vi "Report Save.vi"(4 "Model No.":string, 5 "Report data":string[](array[string])) -> ()   [LabVIEW 2015]
uses:
  <vilib>/Utility/file.llb/Write Delimited Spreadsheet (string).vi
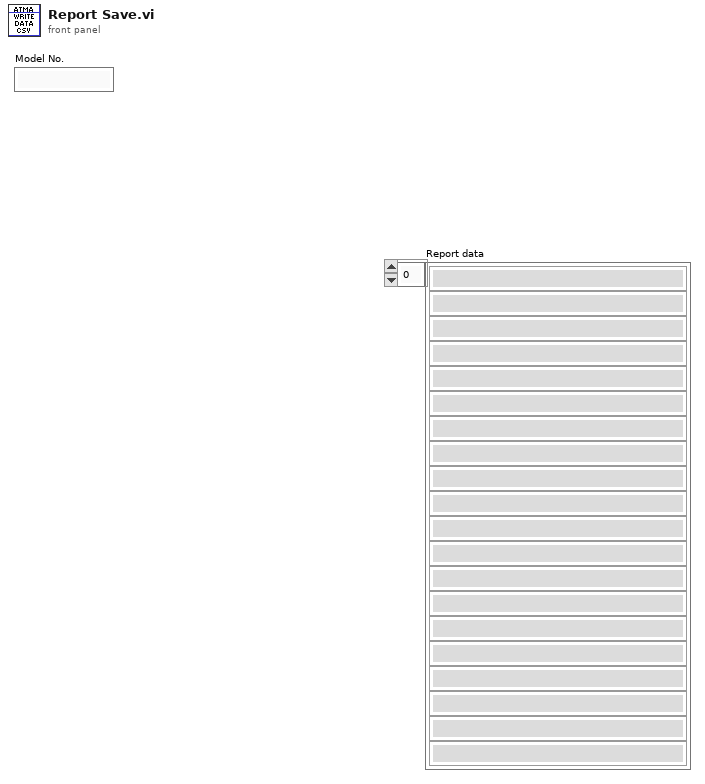
[diagram p1: front panel]
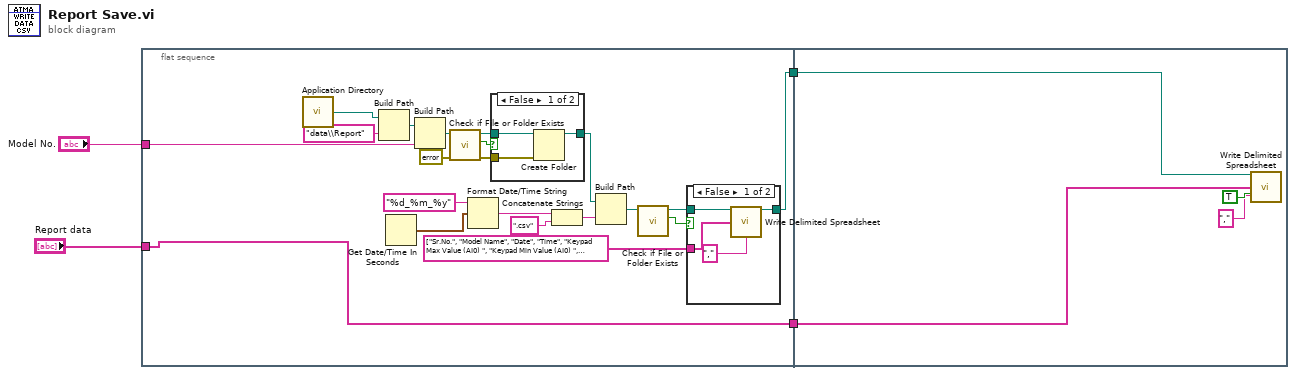
[diagram p0: block diagram]
diagram:
  n1 = flat-sequence {
    tunnel: [w16] -> w4
    tunnel: "Model No." -> [w6]
    tunnel: [w5] -> w2
    tunnel: "Report data" -> [w5]
    tunnel: w4 -> [w36]
    tunnel: w2 -> [w35]
    frame #0 {
      n2 = call <vilib>:"Application Directory.vi"() -> ("Application Directory"=w14:path)
      n3 = Build Path(base path=w14, name or relative path="data\\Report") -> (appended path=w8:path)
      n4 = Get Date/Time In Seconds() -> (seconds since 1Jan1904=w22:timestamp)
      n5 = Build Path(base path=w8, name or relative path=w6) -> (appended path=w7:path)
      n6 = call <vilib>:"Check if File or Folder Exists.vi"("error in (no error)"=errorcluster {"status"=FALSE, "code"=0, "source"=""}, "path"=w7) -> ("error out"=w12:errorcluster, "file or folder exists?"=w10:bool, "dup path"=w13:path)  [unwired: 7 in]
      n7 = Format Date/Time String(time format string (%c)="%d_%m_%y", seconds (now)=w22) -> (date/time string=w20:string)  [unwired: 1 in]
      n8 = case shown="False" w10 {
        tunnel: w13 -> [w28 w29]
        tunnel: [w27 w29] -> w9
        tunnel: w12 -> [w26 _]
        frame False {
          n9 = Create Folder(path (use dialog)=w28, error in=w26) -> (created path=w27:path)  [unwired: 1 in, 2 out]
        }
        frame True {
        }
      }
      n10 = Concatenate Strings(w20, ".csv" ("string")) -> (w18:string)
      n11 = Build Path(base path=w9, name or relative path=w18) -> (appended path=w17:path)
      n12 = call <vilib>:"Check if File or Folder Exists.vi"("path"=w17) -> ("file or folder exists?"=w25:bool, "dup path"=w24:path)  [unwired: 8 in, 1 out]
      n13 = case shown="False" w25 {
        tunnel: [w30 w34] -> w16
        tunnel: w24 -> [w32 w34]
        tunnel: string[] ["Sr.No.", "Model Name", "Date", "Time", "Keypad Max Value (AI0) ", "Keypad Min Value (AI0) ", "Keypad Actual Value (AI0) ", "Keypad Max Value (AI1) ", "Keypad Min Value (AI1) ", "Keypad Actual Value (AI1) ", "Camera Co-ordinate Max Value", "Camera Co-ordinate Min Value", "Camera Co-ordinate Actual Value", "MIC Code", "TFT Display Code", "Status"] -> [w31 _]
        frame False {
          n14 = call-poly <vilib>:"Write Delimited Spreadsheet.vi"("file path (dialog if empty)"=w32, "1D data"=w31, "delimiter (\\t)"="," ("delimiter (\\t)")) -> ("new file path (Not A Path if cancelled)"=w30:path)  [unwired: 11 in, 1 out]
        }
        frame True {
        }
      }
    }
    frame #1 {
      n15 = call-poly <vilib>:"Write Delimited Spreadsheet.vi"("file path (dialog if empty)"=w36, "1D data"=w35, "append to file? (F)"=TRUE, "delimiter (\\t)"="," ("delimiter (\\t)")) -> ()  [unwired: 10 in, 2 out]
    }
  }
